vi "Write Logged Data.vi"(8 "error in (no error)":errorcluster, 10 "Data":T1[](array[typedef]), 11 "PCAP Frame Logger in":refnum<class "PCAP Frame Logger.lvclass">) -> (0 "error out":errorcluster, 3 "PCAP Frame Logger out":refnum<class "PCAP Frame Logger.lvclass">)   [LabVIEW 2020, in "Frame Logging.lvlib" / "PCAP Frame Logger.lvclass"]
uses:
  PCAP Frame Logger.lvclass
  PCAP Frame Logger.lvclass/PCAP Frame Logger.ctl
  <instrlib>/AIM GmbH/_AIM 664/AIM664LV.lvlib
  libpcaplv/libpcaplv.lvlib
  Shared/Frame.ctl
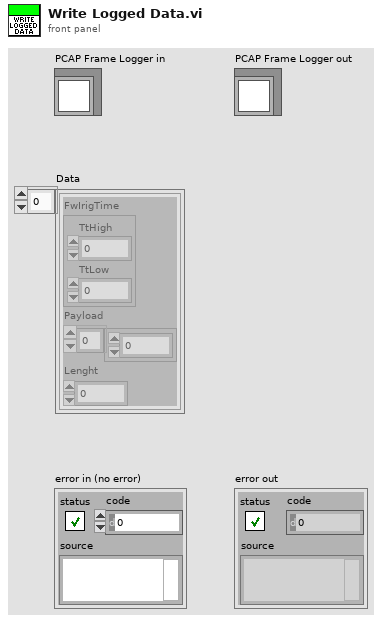
[diagram p1: front panel]
types:
  T1 = typedef "Frame.ctl" = cluster{"FwIrigTime":cluster{"TtHigh":u32, "TtLow":u32}, "Payload":u8[], "Lenght":u32}
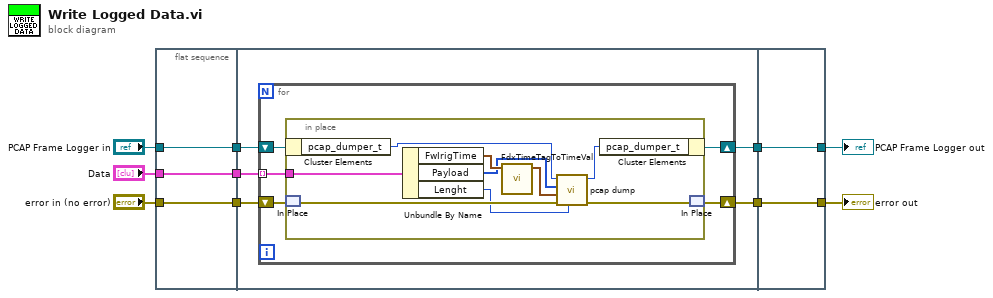
[diagram p0: block diagram]
diagram:
  n1 = flat-sequence {
    tunnel: "Data" -> [w11]
    tunnel: "error in (no error)" -> [w12]
    tunnel: "PCAP Frame Logger in" -> [w13]
    tunnel: [w13] -> w6
    tunnel: [w12] -> w5
    tunnel: [w11] -> w4
    tunnel: w6 -> [w18]
    tunnel: w5 -> [w16]
    tunnel: w4 -> [w14]
    tunnel: [w17] -> w3
    tunnel: [w15] -> w2
    tunnel: [w33] -> w1
    tunnel: [w34] -> w9
    tunnel: w3 -> [w34]
    tunnel: w2 -> [w33]
    frame #0 {
    }
    frame #1 {
      n2 = for {
        shift-right: [w19] -> w17
        shift-left: w18 -> [w21]
        shift-right: [w22] -> w15
        shift-left: w16 -> [w23]
        tunnel: w14 -> [w20] mode=indexing
        n3 = in-place {
          in-place-border: w20 -> [w32]
          n4 = in-place-cluster #1(w21) -> ("pcap_dumper_t"=w25:u64)
          n5 = in-place-match #2(w23) -> (w30:errorcluster)
          n6 = Unbundle By Name(w32) -> ("FwIrigTime"=w31:cluster{"TtHigh":u32, "TtLow":u32}, "Payload"=w28:u8[], "Lenght"=w26:u32)
          n7 = call <instrlib>:"FdxTimeTagToTimeVal.vi"("FwIrigTime"=w31) -> ("timeval"=w27:cluster{"time_t":u64, "useconds_t":u64})  [unwired: 9 in, 1 out]
          n8 = call "pcap dump.vi"("len (0)"=w26, "error in"=w30, "timeval"=w27, "Packet in"=w28, "pcap_dumper_t in"=w25) -> ("error out"=w29:errorcluster, "pcap_dumper_t out"=w24:u64)  [unwired: 5 in]
          n9 = in-place-cluster #1("pcap_dumper_t"=w24) -> (w19:refnum<class "PCAP Frame Logger.lvclass">)
          n10 = in-place-match #2(w29) -> (w22:errorcluster)
        }
      }
    }
    frame #2 {
    }
  }
  "error out" <- w1
  "PCAP Frame Logger out" <- w9
